vi "Read configuration.vi"(8 "error in":errorcluster, 11 "Missing Plugin editor node in":refnum<class "Missing Plugin editor node.lvclass">) -> (0 "error out":errorcluster, 2 "configuration":refnum<class "NISE_CEF_serializable configuration.lvclass">, 3 "Missing Plugin editor node out":refnum<class "Missing Plugin editor node.lvclass">)   [LabVIEW 2014, in "Missing Plugin editor node.lvclass"]
uses:
  Missing Plugin editor node.lvclass
  <vilib>/NI/Configuration Framework/serializable configuration/NISE_CEF_serializable configuration.lvclass
  Missing Plugin editor node.lvclass/Missing Plugin editor node.ctl
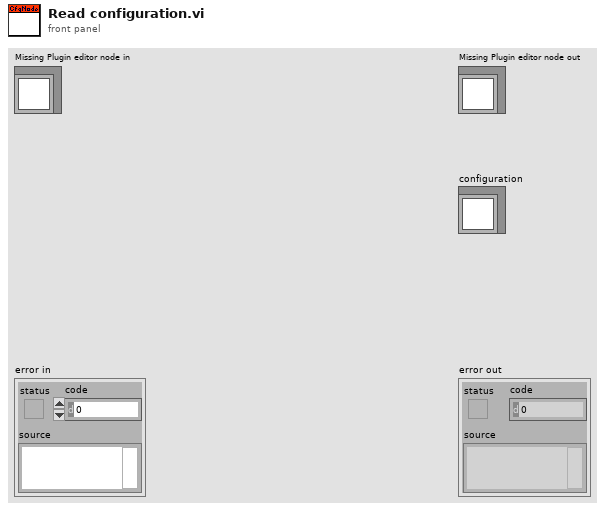
[diagram p1: front panel]
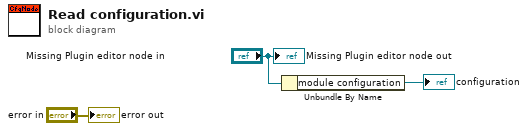
[diagram p0: block diagram]
diagram:
  n1 = Unbundle By Name("Missing Plugin editor node in") -> ("module configuration"=→"configuration":refnum<class "Missing Plugin configuration.lvclass">)
  "error out" <- "error in"
  "Missing Plugin editor node out" <- "Missing Plugin editor node in"
